vi "worker.vi"(9 "timout":i32=-1, 10 "Iterations":i32=6000) -> ()   [LabVIEW 2015]
uses:
  time_logic.vi
  inp.vi
panel:
  out "Numeric":i32
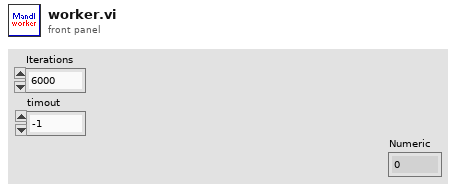
[diagram p1: front panel]
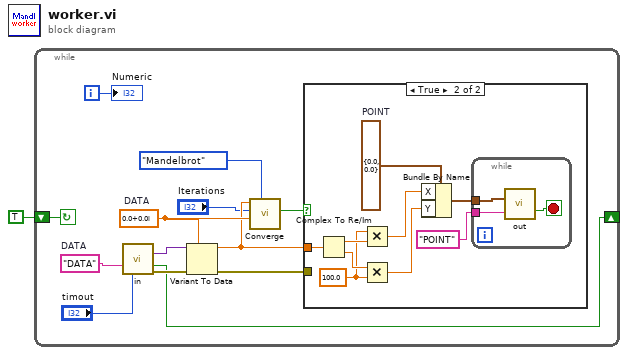
[diagram p0: block diagram]
diagram:
  n1 = while {
    shift-right: [w3] -> _
    shift-left: TRUE ("Valid data") -> [w2]
    i -> [w7]
    stop <- w2 continue-if-true
    w14 = cdb 0.0+0.0i  # DATA
    w6 = "DATA"  # DATA
    n2 = call "in.vi"("Name in"=w6, "timout"="timout") -> ("OUT VARIANT"=w13:variant, "Valid data"=w3:bool, "error out"=w12:errorcluster)  [unwired: 11 in]
    n3 = Variant To Data(error in=w12, type=w14, Variant=w13) -> (data=w11:cdb, error out=w10:errorcluster)
    n4 = call "Converge.vi"("Fractal type"=enum16{"Mandelbrot", "Julia"}."Mandelbrot", "Z0"=w14, "Iterations"="Iterations", "C"=w11) -> ("IN"=w9:bool)  [unwired: 6 in, 1 out]
    n5 = case shown="True" w9 {
      tunnel: w11 -> [_ w23]
      tunnel: w10 -> [_ _]
      frame False {
      }
      frame True {
        w17 = cluster{"X":dbl, "Y":dbl} {"X"=0.0, "Y"=0.0}  # POINT
        w20 = 100.0 ("x")
        n6 = Complex To Re/Im(x + iy=w23) -> (x=w22:dbl, y=w21:dbl)
        n7 = Multiply(x=w20, y=w22) -> (x*y=w19:dbl)
        n8 = Multiply(x=w21, y=w20) -> (x*y=w18:dbl)
        n9 = Bundle By Name(cluster=w17, "X"=w19, "Y"=w18) -> (w15:cluster{"X":dbl, "Y":dbl})
        n10 = while {
          tunnel: "POINT" ("Name in") -> [w24]
          tunnel: w15 -> [w26]
          stop <- w25 stop-if-true
          n11 = call "out.vi"("IN VARIANT"=w26, "Name in"=w24) -> ("Operation Ok"=w25:bool)  [unwired: 12 in, 1 out]
        }
      }
    }
    "Numeric" <- w7
  }
